vi "Vision.vi"() -> ()   [LabVIEW 2020]
uses:
  <vilib>/userDefined/High Color/IMAQdx.ctl
  <vilib>/vision/driver/NI_Vision_Acquisition_Software.lvlib
  <vilib>/vision/NI_Vision_Development_Module.lvlib
panel:
  out "Read String":string
  out "Image":T1(plugin-control)
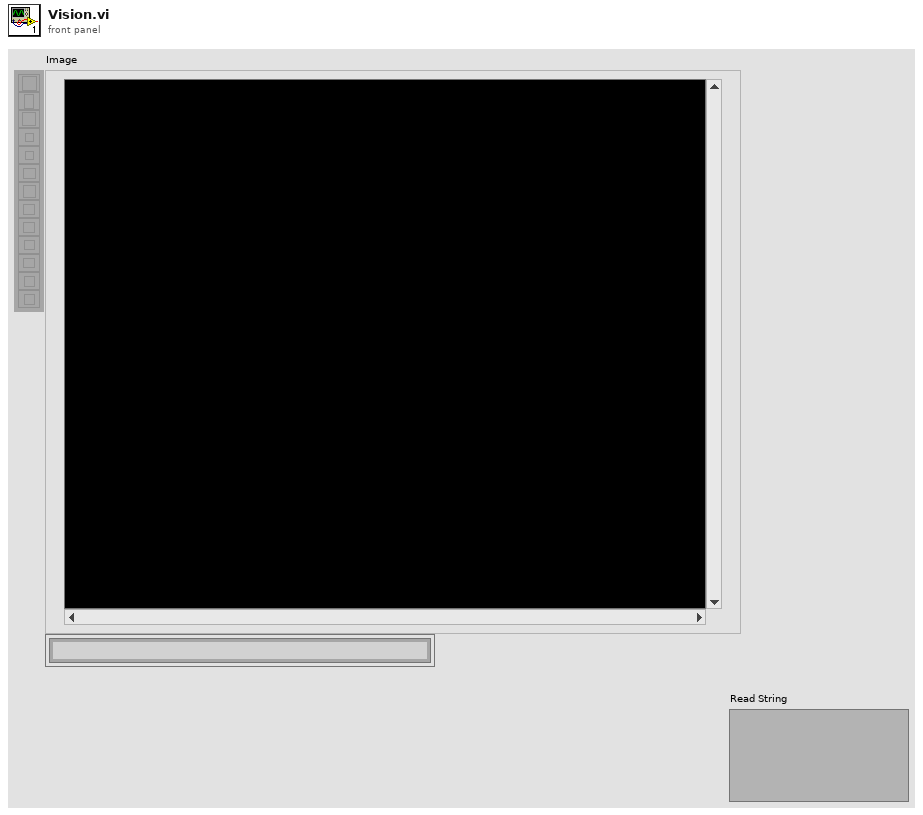
[diagram p1: front panel]
types:
  T1 = typedef "IMAQ Image.ctl" = refnum<image>
  T2 = typedef "IMAQ Rectangle" = cluster{"Left":i32, "Top":i32, "Right":i32, "Bottom":i32, "Rotation":dbl}
  T3 = typedef "IMAQdx.ctl" = refnum<k21>
  T4 = typedef "ROI Descriptor" = cluster{"Global Rectangle":i32[], "Contours":cluster{"ID":enum32{"External", "Internal"}, "Type":u32, "Coordinates":i32[]}[]}
  T5 = typedef "IMAQ OCR Session.ctl" = refnum<k1>
  T6 = cluster{"Global Rectangle":i32[], "Contours":cluster{"ID":enum32{"External", "Internal"}, "Type":u32, "Coordinates":i32[]}[]}
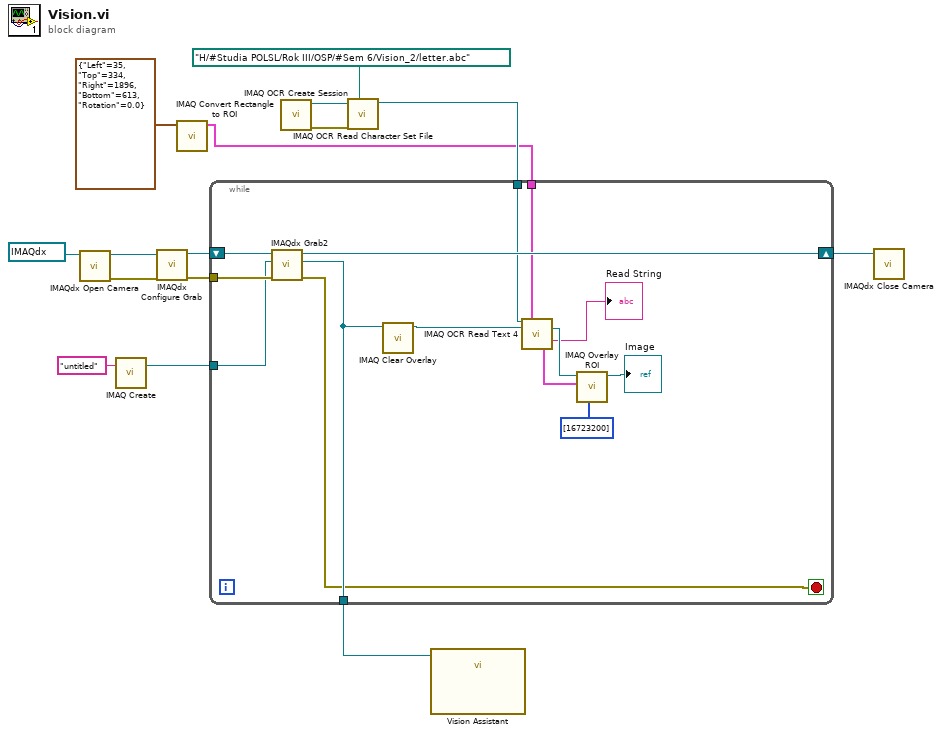
[diagram p0: block diagram]
diagram:
  n1 = call <vilib>:"IMAQdx Open Camera.vi"("Session In"=T3 "cam0") -> ("error out"=w15:errorcluster, "Session Out"=w14:T3)  [unwired: 9 in]
  n2 = call "IMAQ Create"("Image Name"="untitled") -> ("New Image"=w10:T1)  [unwired: 4 in, 1 out]
  n3 = call <vilib>:"IMAQdx Configure Grab.vi"("error in"=w15, "Session In"=w14) -> ("error out"=w12:errorcluster, "Session Out"=w13:T3)  [unwired: 8 in]
  n4 = call "IMAQ Convert Rectangle to ROI"("Rectangle"=T2 {"Left"=35, "Top"=334, "Right"=1896, "Bottom"=613, "Rotation"=0.0}) -> ("ROI Descriptor"=w3:T4)  [unwired: 8 in, 1 out]
  n5 = call "IMAQ OCR Create Session"() -> ("error out"=w6:errorcluster, "IMAQ OCR Session"=w7:T5)  [unwired: 10 in]
  n6 = call "IMAQ OCR Read Character Set File"("File Path"=path "H:/#Studia POLSL/Rok III/OSP/#Sem 6/Vision_2/letter.abc", "error in (no error)"=w6, "IMAQ OCR Session"=w7) -> ("IMAQ OCR Session (dup)"=w4:T5)  [unwired: 6 in, 2 out]
  n7 = while {
    tunnel: w12 -> [w28]
    tunnel: w10 -> [w27]
    shift-right: [w26] -> w9
    shift-left: w13 -> [w29]
    tunnel: w4 -> [w25]
    tunnel: w3 -> [w24]
    tunnel: [w19] -> w2
    stop <- w16 stop-if-true
    n8 = call <vilib>:"IMAQdx Grab2.vi"("error in"=w28, "Image In"=w27, "Session In"=w29) -> ("error out"=w16:errorcluster, "Image Out"=w19:T1, "Session Out"=w26:T3)  [unwired: 5 in, 1 out]
    n9 = call "IMAQ Clear Overlay"("Image"=w19) -> ("Image Out"=w18:T1)  [unwired: 9 in, 1 out]
    n10 = call "IMAQ OCR Read Text 4"("IMAQ OCR Session"=w25, "ROI Descriptor"=w24, "Image"=w18) -> ("Image (dup)"=w23:T1, "Read String"=→"Read String":string, "ROI Bounding Characters"=w21:T6)  [unwired: 6 in, 4 out]
    n11 = call "IMAQ Overlay ROI"("Colors (Green)"=u32[] [16723200], "ROI Descriptor"=w21, "Image"=w23) -> ("Image Out"=→"Image":T1)  [unwired: 7 in, 1 out]
  }
  n12 = call "Vision Assistant"("Image In"=w2) -> ()  [unwired: 25 in, 2 out]
  n13 = call <vilib>:"IMAQdx Close Camera.vi"("Session In"=w9) -> ()  [unwired: 10 in, 1 out]
